vi "Check Pixel Value-2013.vi"() -> ()   [LabVIEW 8.6]
doc: "The Snap VI acquires an image and displays the image in an image control using low-level acquisition VIs. A snap is appropriate for low-speed or single-capture applications in which ease of programming is essential."
uses:
  <vilib>/vision/NI_Vision_Development_Module.lvlib
panel:
  in  "Y Coordinate":i32(slide)
  in  "File Path":path
  in  "stop":bool
  out "Pixel Value (I16)":i16
  in  "X Coordinate":i32(slide)
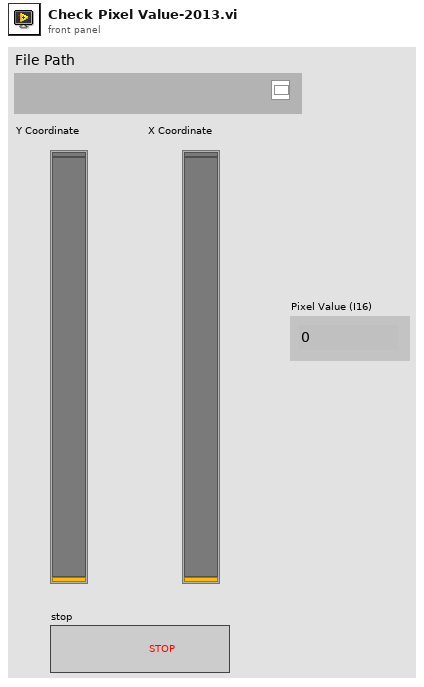
[diagram p1: front panel]
types:
  T1 = typedef "Image Type" = u32
  T2 = typedef "IMAQ Image.ctl" = refnum<image>
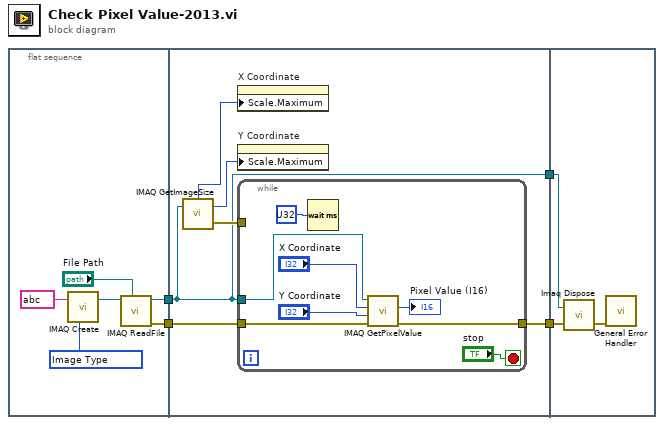
[diagram p0: block diagram]
diagram:
  n1 = flat-sequence {
    tunnel: [w6] -> w4
    tunnel: [w7] -> w3
    tunnel: w4 -> [w16]
    tunnel: w3 -> [w12]
    tunnel: [w15] -> w2
    tunnel: [w12] -> w1
    tunnel: w2 -> [w25]
    tunnel: w1 -> [w26]
    frame #0 {
      w9 = T1 ? items=["Grayscale (U8)", "Grayscale (I16)", "Grayscale (SGL)", "Complex (CSG)", "RGB (U32)", "HSL (U32)", "RGB (U64)", "Grayscale (U16)"] ("Image Type")
      n2 = call "IMAQ Create"("Image Name"=string ?, "Image Type"=w9) -> ("New Image"=w8:T2)  [unwired: 2 in, 2 out]
      n3 = call "IMAQ ReadFile"("File Path"="File Path", "Image"=w8) -> ("error out"=w6:errorcluster, "Image Out"=w7:T2)  [unwired: 5 in, 3 out]
    }
    frame #1 {
      n4 = call "IMAQ GetImageSize"("Image"=w12) -> ("Y Resolution"=w14:i32, "X Resolution"=w11:i32, "error out"=w13:errorcluster)  [unwired: 3 in]
      n5 = property on="X Coordinate" class="Slide (strict)"("Scale.Maximum"=w11) -> ()  [unwired: 2 in, 2 out]
      n6 = property on="Y Coordinate" class="Slide (strict)"("Scale.Maximum"=w14) -> ()  [unwired: 2 in, 2 out]
      n7 = while {
        tunnel: w16 -> [w24]
        tunnel: [w23] -> w15
        tunnel: w12 -> [w20]
        tunnel: w13 -> [_]
        stop <- "stop" stop-if-true
        n8 = Wait (ms)(milliseconds to wait=u32 ?) -> ()  [unwired: 1 out]
        n9 = call "IMAQ GetPixelValue"("Image"=w20, "X Coordinate"="X Coordinate", "Y Coordinate"="Y Coordinate", "error in (no error)"=w24) -> ("Pixel Value (I16)"=→"Pixel Value (I16)":i16, "error out"=w23:errorcluster)  [unwired: 2 in, 3 out]
      }
    }
    frame #2 {
      n10 = call "Imaq Dispose"("Image"=w26, "error in (no error)"=w25) -> ("error out"=w27:errorcluster)  [unwired: 4 in]
      n11 = call <vilib>:"General Error Handler.vi"("error in (no error)"=w27) -> ()  [unwired: 1 in, 14 out]
    }
  }
